vi "Stime.vi"(3 "current time":timestamp) -> (0 "time stamp":timestamp, 1 "x != y?":bool)   [LabVIEW 2013]
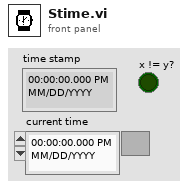
[diagram p1: front panel]
types:
  T1 = typedef "LVDateTimeRec.ctl" = cluster{"fractional second":dbl, "second":i32, "minute":i32, "hour":i32, "day of month":i32, "month":i32, "year":i32, "day of week":i32, "day of year":i32, "DST":i32}
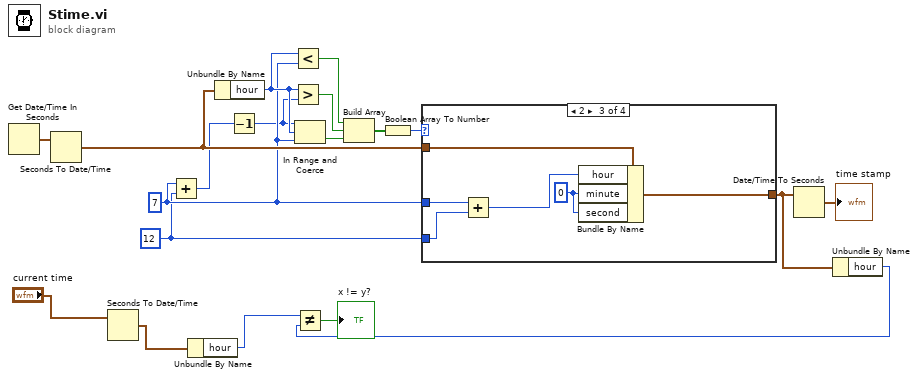
[diagram p0: block diagram]
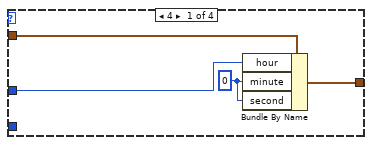
[diagram p2: hidden frame]
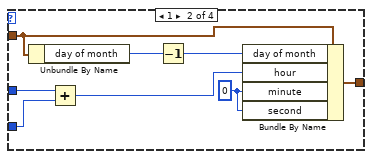
[diagram p3: hidden frame]
diagram:
  w9 = 12 ("y")
  w10 = 7 ("y")
  n1 = Get Date/Time In Seconds() -> (seconds since 1Jan1904=w18:timestamp)
  n2 = Seconds To Date/Time(time stamp (now)=w18) -> (date time rec=w12:T1)  [unwired: 1 in]
  n3 = Seconds To Date/Time(time stamp (now)="current time") -> (date time rec=w5:T1)  [unwired: 1 in]
  n4 = Add(x=w10, y=w9) -> (x+y=w8:i32)
  n5 = Unbundle By Name(w5) -> ("hour"=w4:i32)
  n6 = Unbundle By Name(w12) -> ("hour"=w11:i32)
  n7 = Decrement(x=w8) -> (x-1=w7:i32)
  n8 = Less?(x=w11, y=w10) -> (x < y?=w17:bool)
  n9 = Greater?(x=w11, y=w7) -> (0:w16:bool)
  n10 = In Range and Coerce(upper limit=w7, x=w11, lower limit=w10) -> (In Range?=w15:bool)  [unwired: 1 out]
  n11 = Build Array(w17, w16, w15) -> (w14:bool[])
  n12 = Boolean Array To Number(Boolean array=w14) -> (number=w13:u32)
  n13 = case shown="2" w13 {
    tunnel: w12 -> [w22 w29 w36 w38]
    tunnel: [w21 w31 w35 w38] -> w3
    tunnel: w10 -> [w20 w26 w34 _]
    tunnel: w9 -> [_ w25 w33 _]
    frame 4 {
      w23 = 0 ("minute")
      n14 = Bundle By Name(cluster=w22, "hour"=w20, "minute"=w23, "second"=w23) -> (w21:T1)
    }
    frame 1 {
      w30 = 0 ("minute")
      n15 = Unbundle By Name(w29) -> ("day of month"=w28:i32)
      n16 = Add(x=w26, y=w25) -> (x+y=w24:i32)
      n17 = Decrement(x=w28) -> (x-1=w27:i32)
      n18 = Bundle By Name(cluster=w29, "day of month"=w27, "hour"=w24, "minute"=w30, "second"=w30) -> (w31:T1)
    }
    frame 2 {
      w37 = 0 ("minute")
      n19 = Add(x=w34, y=w33) -> (x+y=w32:i32)
      n20 = Bundle By Name(cluster=w36, "hour"=w32, "minute"=w37, "second"=w37) -> (w35:T1)
    }
    frame Default {
    }
  }
  n21 = Date/Time To Seconds(2:w3) -> (0:→"time stamp":timestamp)  [unwired: 1 in]
  n22 = Unbundle By Name(w3) -> ("hour"=w2:i32)
  n23 = Not Equal?(x=w4, y=w2) -> (x != y?=→"x != y?":bool)
